vi "X Cubed.vi"(1 "X":dbl) -> (0 "X^3":dbl)   [LabVIEW 2016]
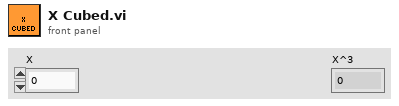
[diagram p1: front panel]
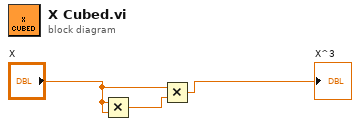
[diagram p0: block diagram]
diagram:
  n1 = Multiply(x="X", y="X") -> (x*y=w3:dbl)
  n2 = Multiply(x="X", y=w3) -> (x*y=→"X^3":dbl)
